vi "generate waveform.vi"(11 "Status":T1 {"Setting"."X Pos." scale=-2.0..2.0; "Setting"."Y Pos." scale=-2.0..2.0}) -> (2 "sample number":i32, 3 "波形图":waveform(dbl)[](graph))   [LabVIEW 2013]
uses:
  init & communication/init-status.ctl
  init & communication/Setting.ctl
  init & communication/event-package.ctl
  init & communication/Event1.ctl
  init & communication/data-package.ctl
  init & communication/Event.ctl
panel:
  out "大小 2":i32=20
  out "大小":i32=20
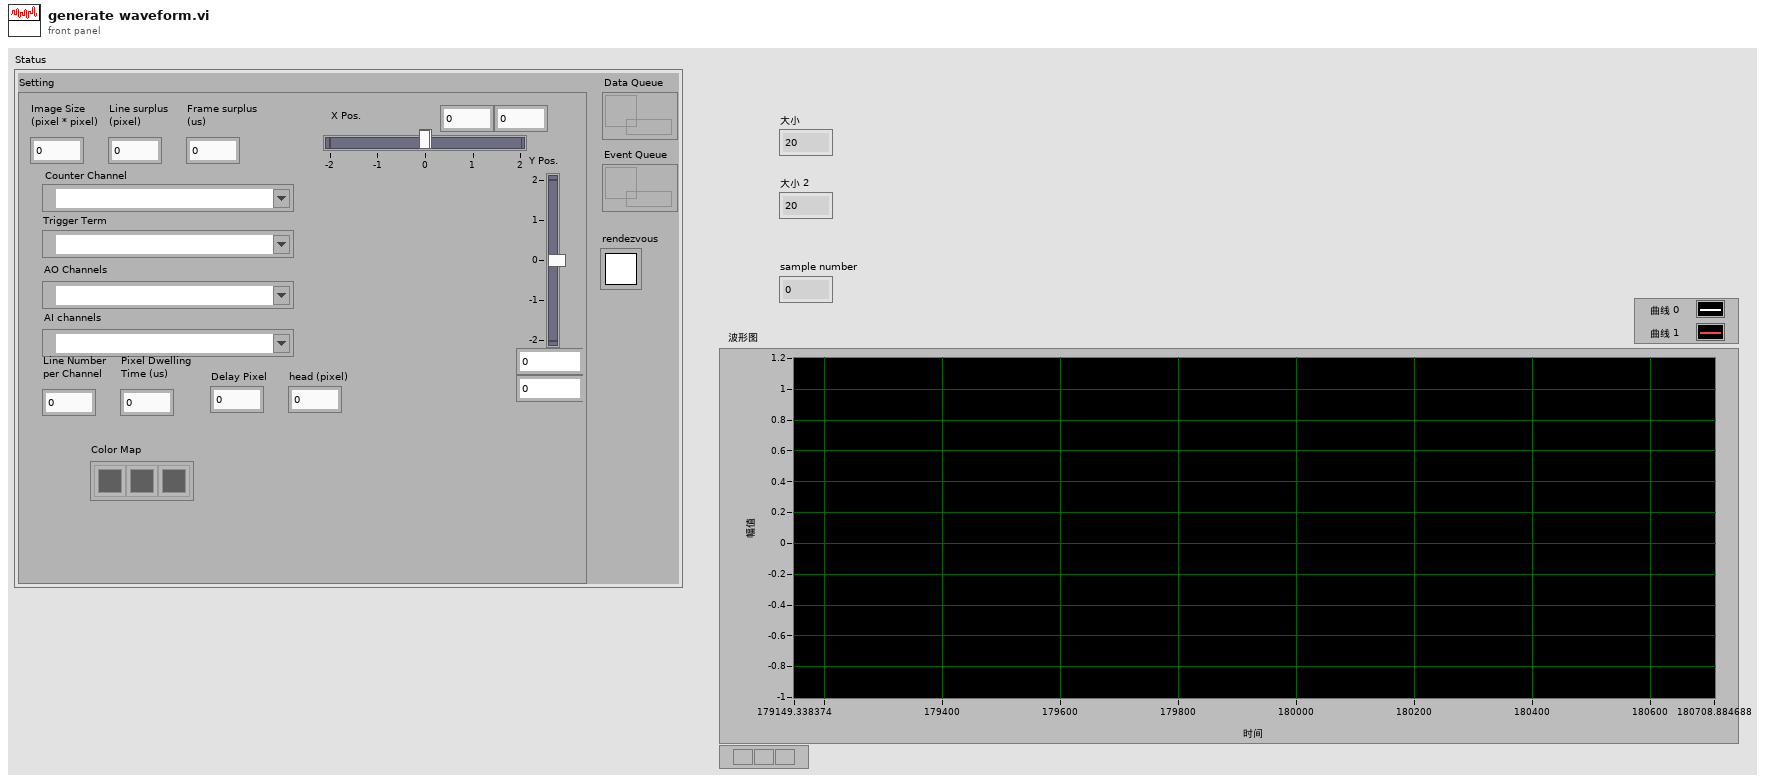
[diagram p1: front panel]
types:
  T1 = typedef "init-status.ctl" = cluster{"Setting":T2, "Event Queue":refnum<queue>, "Data Queue":refnum<queue>, "rendezvous":T3}
  T2 = typedef "Setting.ctl" = cluster{"Image Size\n(pixel * pixel)":i32, "Counter Channel":tag, "Trigger Term":tag, "AO Channels":tag, "Y Pos.":cluster{dbl, dbl}, "X Pos.":cluster{dbl, dbl}, "Line surplus\n(pixel)":i32, "Frame surplus\n(us)":i32, "AI channels":tag, "Line Number\nper Channel":i32, "Delay Pixel":i32, "Pixel Dwelling\nTime (us)":i32, "Color Map":u32[], "head (pixel)":i32}
  T3 = typedef "Rendezvous RefNum" = refnum<k1>
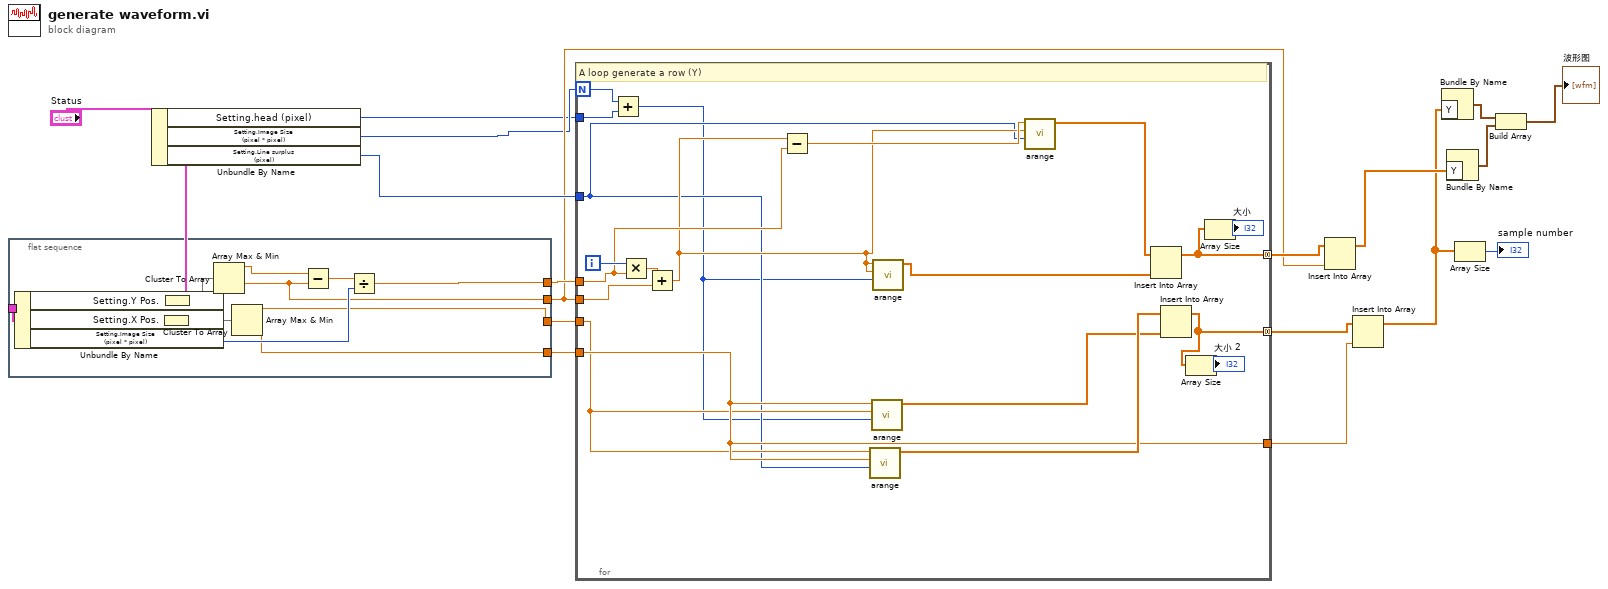
[diagram p0: block diagram]
diagram:
  n1 = flat-sequence {
    tunnel: "Status" -> [w29]
    tunnel: [w21] -> w16
    tunnel: [w20] -> w4
    tunnel: [w19] -> w15
    tunnel: [w18] -> w3
    frame #0 {
      n2 = Unbundle By Name(w29) -> ("Setting.Y Pos."=w28:cluster{dbl, dbl}, "Setting.X Pos."=w27:cluster{dbl, dbl}, "Setting.Image Size\n(pixel * pixel)"=w22:i32)
      n3 = Cluster To Array(cluster=w27) -> (array=w25:dbl[])
      n4 = Cluster To Array(cluster=w28) -> (array=w26:dbl[])
      n5 = Array Max & Min(array=w26) -> (max value=w23:dbl, min value=w20:dbl)  [unwired: 2 out]
      n6 = Array Max & Min(array=w25) -> (max value=w18:dbl, min value=w19:dbl)  [unwired: 2 out]
      n7 = Subtract(x=w23, y=w20) -> (x-y=w24:dbl)
      n8 = Divide(x=w24, y=w22) -> (x/y=w21:dbl)
    }
  }
  n9 = Unbundle By Name("Status") -> ("Setting.head (pixel)"=w1:i32, "Setting.Image Size\n(pixel * pixel)"=w2:i32, "Setting.Line surplus\n(pixel)"=w14:i32)
  n10 = for {
    N: w2 -> [w31]
    tunnel: w16 -> [w41]
    tunnel: w4 -> [w47]
    tunnel: w15 -> [w39]
    tunnel: w14 -> [w33]
    tunnel: [w46] -> w8 mode=concatenating
    tunnel: [w43] -> w9 mode=concatenating
    tunnel: [w39] -> w5
    tunnel: w3 -> [w38]
    tunnel: w1 -> [w32]
    i -> [w49]
    # "A loop generate a row (Y)"
    n11 = Add(x=w31, y=w32) -> (x+y=w30:i32)
    n12 = Multiply(x=w49, y=w41) -> (x*y=w48:dbl)
    n13 = Add(x=w48, y=w47) -> (x+y=w34:dbl)
    n14 = Subtract(x=w34, y=w41) -> (x-y=w35:dbl)
    n15 = call "arange.vi"("Number of pixels"=w33, "end"=w39, "begin"=w38) -> ("数组"=w40:dbl[])  [unwired: 8 in]
    n16 = call "arange.vi"("Number of pixels"=w30, "end"=w38, "begin"=w39) -> ("数组"=w37:dbl[])  [unwired: 8 in]
    n17 = call "arange.vi"("Number of pixels"=w30, "end"=w34, "begin"=w34) -> ("数组"=w36:dbl[])  [unwired: 8 in]
    n18 = call "arange.vi"("Number of pixels"=w33, "end"=w34, "begin"=w35) -> ("数组"=w42:dbl[])  [unwired: 8 in]
    n19 = Insert Into Array(array=w42, new element=w36) -> (w46:dbl[])  [unwired: 1 in]
    n20 = Insert Into Array(array=w40, new element=w37) -> (w43:dbl[])  [unwired: 1 in]
    n21 = Array Size(array=w43) -> (size(s)=→"大小 2":i32)
    n22 = Array Size(array=w46) -> (size(s)=→"大小":i32)
  }
  n23 = Insert Into Array(array=w8, new element=w4) -> (w7:dbl[])  [unwired: 1 in]
  n24 = Insert Into Array(array=w9, new element=w5) -> (w6:dbl[])  [unwired: 1 in]
  n25 = Bundle By Name("Y"=w6) -> (w12:waveform(dbl))  [unwired: 1 in]
  n26 = Bundle By Name("Y"=w7) -> (w11:waveform(dbl))  [unwired: 1 in]
  n27 = Array Size(array=w6) -> (size(s)=→"sample number":i32)
  n28 = Build Array(w12, w11) -> (→"波形图":waveform(dbl)[])
